vi "Convert Metadata to String.vi"(9 "Date Updated":timestamp, 10 "Date Created":timestamp, 11 "Resolutions":cluster{"Width":i16, "Height":i16}[](array[cluster])) -> (3 "Metdata":string)   [LabVIEW 2020, in "MacroAssert.lvlib"]
doc: "Converts various metadata elements into a single string to be saved to an INI."
uses:
  MacroAssert.lvlib
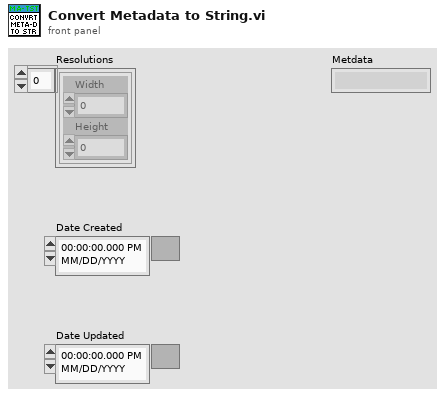
[diagram p1: front panel]
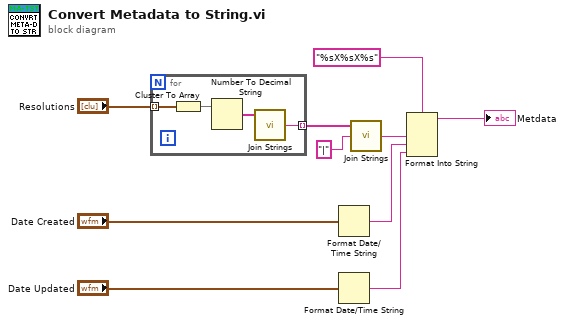
[diagram p0: block diagram]
diagram:
  n1 = for {
    tunnel: "Resolutions" -> [w14] mode=indexing
    tunnel: [w11] -> w9 mode=indexing
    n2 = Cluster To Array(cluster=w14) -> (array=w13:i16[])
    n3 = Number To Decimal String(number=w13) -> (decimal integer string=w12:string[])  [unwired: 1 in]
    n4 = call <vilib>:"Join Strings.vi"("Strings In"=w12) -> ("String"=w11:string)  [unwired: 2 in]
  }
  n5 = Format Date/Time String(seconds (now)="Date Created") -> (date/time string=w3:string)  [unwired: 2 in]
  n6 = Format Date/Time String(seconds (now)="Date Updated") -> (date/time string=w2:string)  [unwired: 2 in]
  n7 = call <vilib>:"Join Strings.vi"("Separator (,)"="|", "Strings In"=w9) -> ("String"=w4:string)  [unwired: 1 in]
  n8 = Format Into String(format string="%sX%sX%s", w4, w3, w2) -> (resulting string=→"Metdata":string)  [unwired: 2 in, 1 out]
